vi "Boolean String to Boolean Array.vi"(10 "Diagnostic Data":string[](array[string])) -> (2 "Diagostic Array Out":bool[][](array[boolean]))   [LabVIEW 2020]
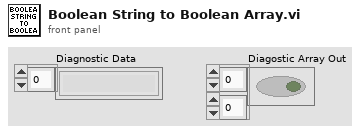
[diagram p1: front panel]
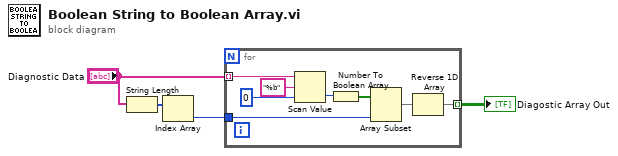
[diagram p0: block diagram]
diagram:
  n1 = String Length(string="Diagnostic Data") -> (length=w1:i32[])
  n2 = Index Array(array=w1) -> (element=w2:i32)  [unwired: 1 in]
  n3 = for {
    tunnel: "Diagnostic Data" -> [w9] mode=indexing
    tunnel: [w6] -> w4 mode=indexing
    tunnel: w2 -> [w5]
    n4 = Scan Value(string=w9, format string="%b", default (0 dbl)=u16 0) -> (value=w10:u16)  [unwired: 1 out]
    n5 = Number To Boolean Array(number=w10) -> (Boolean array=w8:bool[])
    n6 = Array Subset(array=w8, length=w5) -> (w7:bool[])  [unwired: 1 in]
    n7 = Reverse 1D Array(array=w7) -> (reversed array=w6:bool[])
  }
  "Diagostic Array Out" <- w4
